vi "Manual Scale.vi"(8 "error in (no error)":errorcluster, 9 "Secs/div":dbl, 10 "V/div":T1, 11 "DPO4104 in":refnum<class "DPO4104.lvclass">) -> (0 "error out":errorcluster, 3 "DPO4104 out":refnum<class "DPO4104.lvclass">)   [LabVIEW 2018, in "DPO4104.lvlib" / "DPO4104.lvclass"]
doc: "This Overrride is used to manually adjust the scale of the instrument."
uses:
  DPO4104.lvclass
  PPLs/Oscilloscope/Parent/Oscilloscope.lvlibp/Custom Controls/Volts per Division.ctl
  PPLs/Oscilloscope/Parent/Oscilloscope.lvlibp/Custom Controls/Analog Channels.ctl
  PPLs/Oscilloscope/Parent/Oscilloscope.lvlibp/Oscilloscope.lvclass
  C:/Projects/LabVIEW/PPLs/Oscilloscope/Parent/Oscilloscope.lvlibp/Oscilloscope.lvclass
  PPLs/Oscilloscope/Parent/Oscilloscope.lvlibp
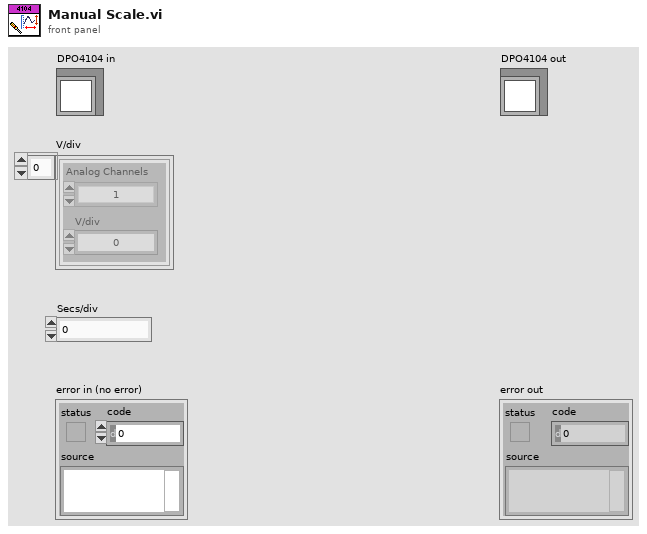
[diagram p1: front panel]
types:
  T1 = typedef "Oscilloscope.lvlibp/Volts per Division.ctl" = cluster{"Analog Channels":T2, "V/div":dbl}[]
  T2 = typedef "Oscilloscope.lvlibp/Analog Channels.ctl" = enum16{"1", "2", "3", "4", "5", "6", "7", "8", "9", "10", "11", "12", "13", "14", "15", "16"}
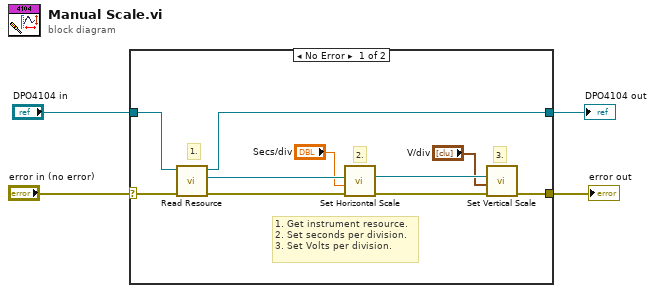
[diagram p0: block diagram]
diagram:
  n1 = case shown="No Error" "error in (no error)" {
    selector: "error in (no error)" -> [w12 w16]
    tunnel: [w6 w16] -> w3
    tunnel: [w13 w15] -> w2
    tunnel: "DPO4104 in" -> [w14 w15]
    frame No Error {
      # "1. Get instrument resource.\n2. Set seconds per division.\n3. Set Volts per division."
      # "3."
      # "2."
      # "1."
      n2 = call "Read Resource.vi"("error in (no error)"=w12, "Oscilloscope in"=w14) -> ("error out"=w11:errorcluster, "Resource"=w10:refnum<visa-resource-name>, "Oscilloscope out"=w13:refnum<class "DPO4104.lvclass">)  [unwired: 7 in]
      n3 = call "Set Horizontal Scale.vi"("error in (no error)"=w11, "Secs/div"="Secs/div", "VISA resource name"=w10) -> ("error out"=w7:errorcluster, "VISA resource name out"=w8:refnum<visa-resource-name>)  [unwired: 7 in]
      n4 = call "Set Vertical Scale.vi"("error in (no error)"=w7, "Channels V/div"="V/div", "VISA resource name"=w8) -> ("error out"=w6:errorcluster)  [unwired: 7 in, 1 out]
    }
    frame Error {
    }
  }
  "error out" <- w3
  "DPO4104 out" <- w2
